vi "Instrument Manager Loop.vi"(8 "System Control":refnum<queue>, 11 "Instrument Manager":refnum<queue>) -> (0 "error out":errorcluster)   [LabVIEW 2020, in "Omega Platinum Series Plugin.lvlib" / "Instrument Manager.lvlib"]
uses:
  Instrument Manager/Instrument Manager.lvlib
  support/Message Queue/Message Cluster.ctl
  Instrument Manager/Instrument State.ctl
  <vilib>/Utility/error.llb/Error Cluster From Error Code.vi
  <vilib>/ErrorRing/Error Ring.xnode
  support/Message Queue/Message Queue.lvlib
  Omega Platinum Series Plugin.lvlib
  <instrlib>/Omega Platinum Series/Omega Platinum Series.lvlib
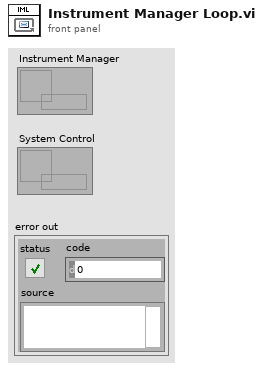
[diagram p1: front panel]
types:
  T1 = typedef "Omega Platinum Series Plugin.lvlib/Instrument Manager.lvlib/Instrument State.ctl" = cluster{"VISA Resource":refnum<visa-resource-name>, "Setpoint":dbl, "Running":bool, "Running Since":timestamp, "Data Point":cluster{"Time Stamp":timestamp, "Value":dbl}, "Sampling Rate (sec/sample)":dbl}
  T2 = typedef "Omega Platinum Series.lvlib/System State.ctl" = enum16{"LOAD", "IDLE", "INPUT_ADJUST", "CONTROL_ADJUST", "MODIFY", "WAIT", "RUN", "STANDBY", "STOP", "PAUSE", "FAULT", "SHUTDOWN", "AUTOTUNE"}
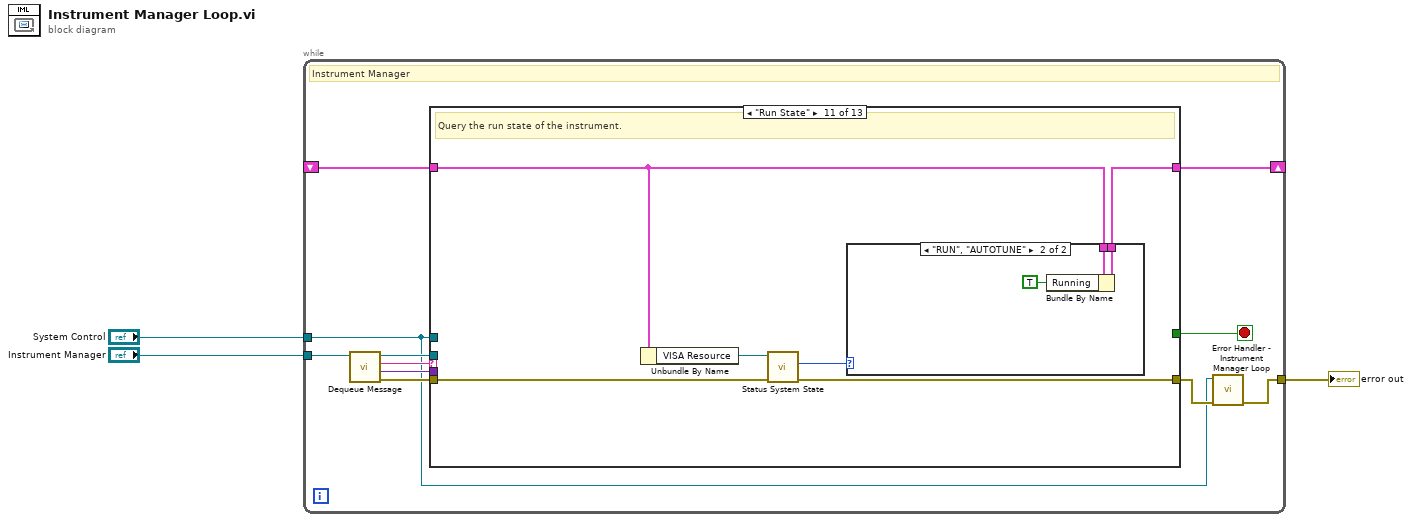
[diagram p0: block diagram]
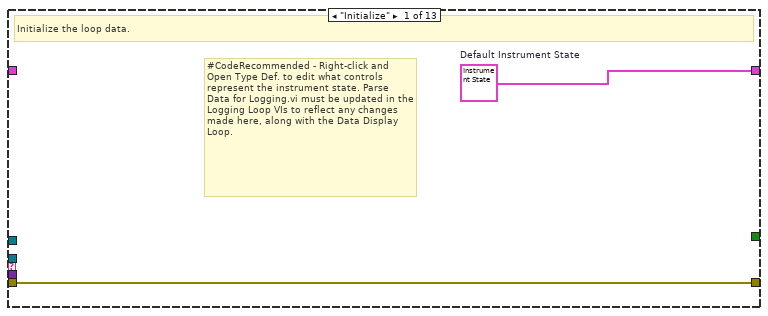
[diagram p2: hidden frame]
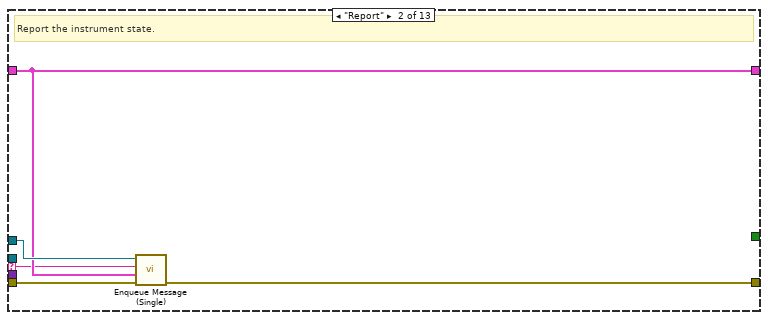
[diagram p3: hidden frame]
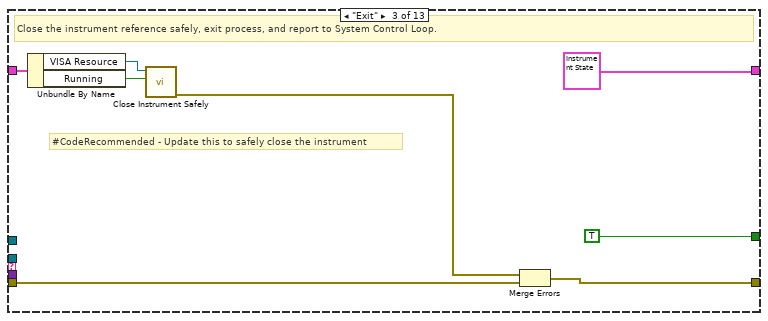
[diagram p4: hidden frame]
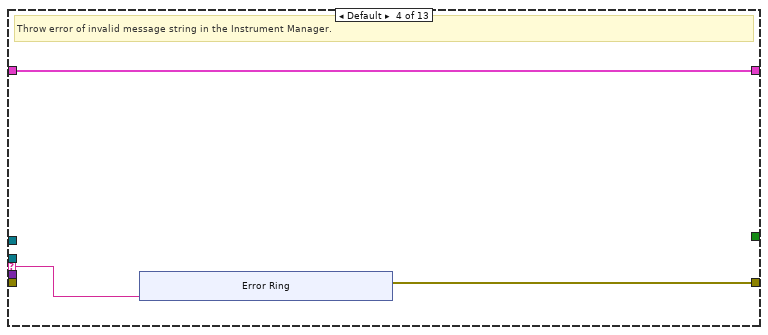
[diagram p5: hidden frame]
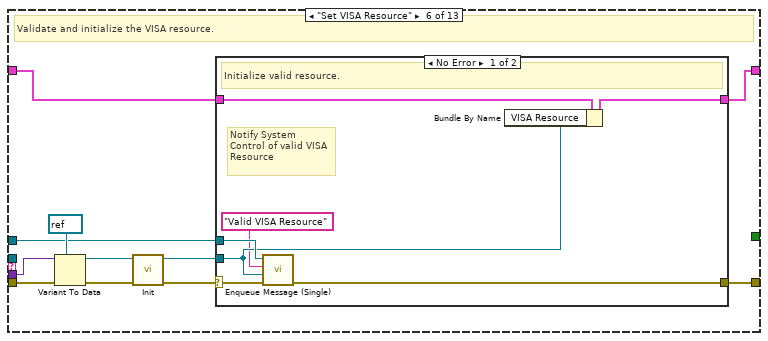
[diagram p7: hidden frame]
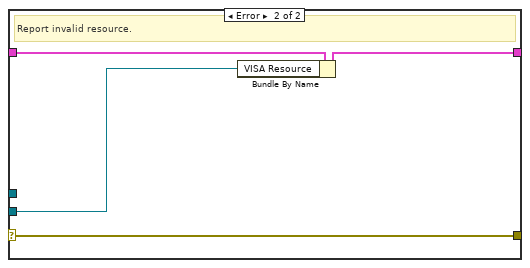
[diagram p8: hidden frame]
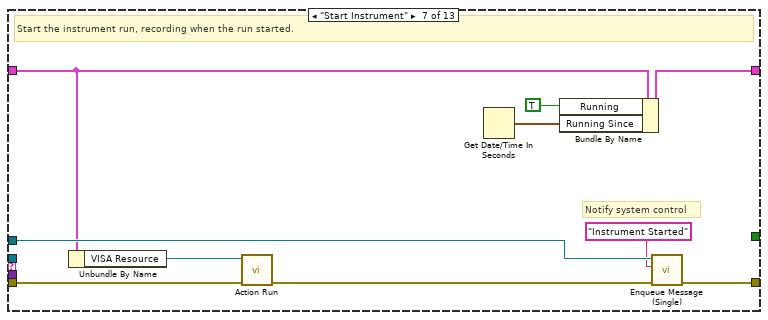
[diagram p9: hidden frame]
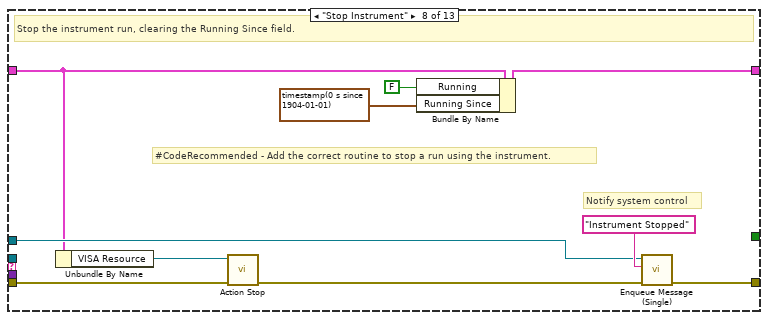
[diagram p10: hidden frame]
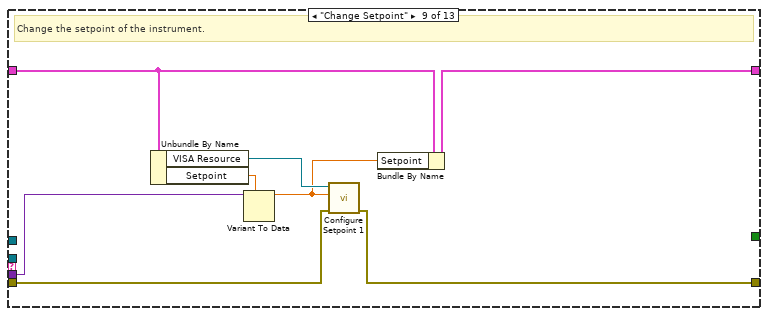
[diagram p11: hidden frame]
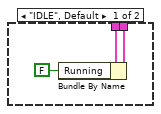
[diagram p13: hidden frame]
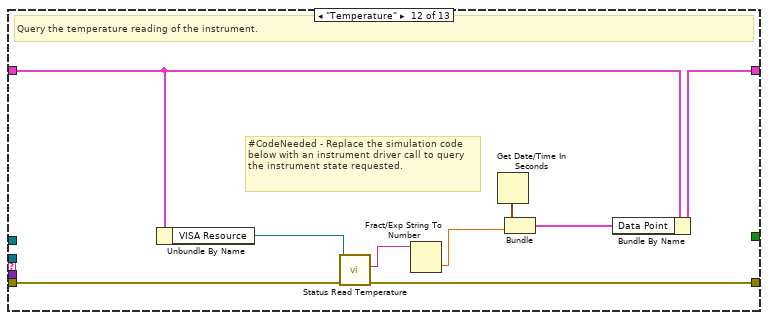
[diagram p14: hidden frame]
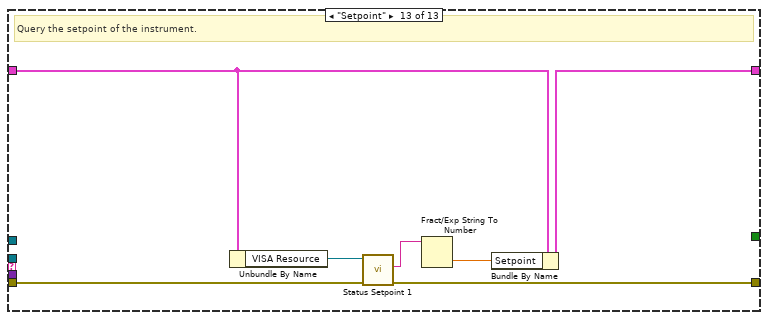
[diagram p15: hidden frame]
diagram:
  n1 = while {
    tunnel: "Instrument Manager" -> [w14]
    tunnel: "System Control" -> [w5]
    tunnel: [w8] -> w1
    shift-right: [w7] -> _
    shift-left: _ -> [w4]
    stop <- w6 stop-if-true
    # "Instrument Manager"
    n2 = call "Dequeue Message.vi"("Message Queue"=w14) -> ("error out"=w10:errorcluster, "Message Data"=w11:variant, "Message"=w13:string, "dup Message Queue"=w12:refnum<queue>)  [unwired: 7 in]
    n3 = case shown="\"Run State\"" w13 {
      selector: w13 -> [_ w17 _ w31 _ _ _ _ _ _ _ _ _]
      tunnel: w12 -> [_ _ _ _ _ _ _ _ _ _ _ _ _]
      tunnel: w5 -> [_ w20 _ _ _ w42 w72 w81 _ _ _ _ _]
      tunnel: w11 -> [_ _ _ _ _ w49 _ _ w90 _ _ _ _]
      tunnel: w10 -> [w15 w21 w24 _ w40 w48 w65 w76 w87 w93 w99 w109 w121]
      tunnel: [w15 w19 w23 w30 w40 w52 w73 w83 w86 w93 w98 w108 w120] -> w9
      tunnel: w4 -> [_ w18 w29 w32 w41 w51 w67 w74 w89 w92 w94 w111 w119]
      tunnel: [w16 w18 T1 {"VISA Resource"="", "Setpoint"=0.0, "Running"=FALSE, "Running Since"=timestamp(0 s since 1904-01-01), "Data Point"={"Time Stamp"=timestamp(0 s since 1904-01-01), "Value"=0.0}, "Sampling Rate (sec/sample)"=0.0} w32 w41 w50 w70 w80 w91 w92 w95 w114 w117] -> w7
      tunnel: [_ _ TRUE _ _ _ _ _ _ _ _ _ _] -> w6
      frame "Initialize" {
        w16 = T1 {"VISA Resource"="", "Setpoint"=0.0, "Running"=FALSE, "Running Since"=timestamp(0 s since 1904-01-01), "Data Point"={"Time Stamp"=timestamp(0 s since 1904-01-01), "Value"=0.0}, "Sampling Rate (sec/sample)"=0.0}  # Default Instrument State
        # "#CodeRecommended - Right-click and Open Type Def. to edit what controls represent the instrument state. Parse Data for Logging.vi must be updated in the Logging Loop VIs to reflect any changes made here, along with the Data Display Loop."
        # "Initialize the loop data."
      }
      frame "Report" {
        # "Report the instrument state."
        n4 = call "Enqueue Message (Single).vi"("error in (no error)"=w21, "Message Data"=w18, "Message"=w17, "Message Queue"=w20) -> ("error out"=w19:errorcluster)  [unwired: 6 in, 1 out]
      }
      frame "Exit" {
        # "#CodeRecommended - Update this to safely close the instrument"
        # "Close the instrument reference safely, exit process, and report to System Control Loop."
        n5 = Unbundle By Name(w29) -> ("VISA Resource"=w27:refnum<visa-resource-name>, "Running"=w28:bool)
        n6 = call "Close Instrument Safely.vi"("Running (F)"=w28, "VISA Refnum in"=w27) -> ("error out"=w22:errorcluster)  [unwired: 9 in]
        n7 = Merge Errors(w22, w24) -> (w23:errorcluster)
      }
      frame Default {
        # "Throw error of invalid message string in the Instrument Manager."
        n8 = xnode "Error Ring"("parameter 0"=w31) -> ("error out"=w30:errorcluster)
      }
      frame "--- Copy This Frame ---" {
        # "Copy this frame and add responses to instrument specific messages."
      }
      frame "Set VISA Resource" {
        # "Validate and initialize the VISA resource."
        n9 = Variant To Data(error in=w48, type=refnum<visa-resource-name> refnum, Variant=w49) -> (data=w46:refnum<visa-resource-name>, error out=w47:errorcluster)
        n10 = call "Init.vi"("error in (no error)"=w47, "VISA resource in"=w46) -> ("error out"=w43:errorcluster, "VISA resource out"=w44:refnum<visa-resource-name>)  [unwired: 8 in]
        n11 = case shown="No Error" w43 {
          selector: w43 -> [w58 w60]
          tunnel: w44 -> [w55 w61]
          tunnel: [w57 w60] -> w52
          tunnel: w51 -> [w59 w63]
          tunnel: [w53 w62] -> w50
          tunnel: w42 -> [w56 _]
          frame No Error {
            # "Notify System Control of valid VISA Resource"
            # "Initialize valid resource."
            n12 = call "Enqueue Message (Single).vi"("error in (no error)"=w58, "Message Data"=w55, "Message"="Valid VISA Resource", "Message Queue"=w56) -> ("error out"=w57:errorcluster)  [unwired: 6 in, 1 out]
            n13 = Bundle By Name(cluster=w59, "VISA Resource"=w55) -> (w53:T1)
          }
          frame Error {
            # "Report invalid resource."
            n14 = Bundle By Name(cluster=w63, "VISA Resource"=w61) -> (w62:T1)
          }
        }
      }
      frame "Start Instrument" {
        # "Notify system control"
        # "Start the instrument run, recording when the run started."
        n15 = Unbundle By Name(w67) -> ("VISA Resource"=w66:refnum<visa-resource-name>)
        n16 = call <instrlib>:"Action Run.vi"("error in (no error)"=w65, "VISA resource name (in)"=w66) -> ("error out"=w64:errorcluster)  [unwired: 7 in, 2 out]
        n17 = Get Date/Time In Seconds() -> (seconds since 1Jan1904=w68:timestamp)
        n18 = Bundle By Name(cluster=w67, "Running"=TRUE, "Running Since"=w68) -> (w70:T1)
        n19 = call "Enqueue Message (Single).vi"("error in (no error)"=w64, "Message"="Instrument Started", "Message Queue"=w72) -> ("error out"=w73:errorcluster)  [unwired: 7 in, 1 out]
      }
      frame "Stop Instrument" {
        # "Notify system control"
        # "#CodeRecommended - Add the correct routine to stop a run using the instrument."
        # "Stop the instrument run, clearing the Running Since field."
        n20 = Unbundle By Name(w74) -> ("VISA Resource"=w77:refnum<visa-resource-name>)
        n21 = call <instrlib>:"Action Stop.vi"("error in (no error)"=w76, "VISA resource name (in)"=w77) -> ("error out"=w75:errorcluster)  [unwired: 7 in, 2 out]
        n22 = Bundle By Name(cluster=w74, "Running"=FALSE, "Running Since"=timestamp(0 s since 1904-01-01)) -> (w80:T1)
        n23 = call "Enqueue Message (Single).vi"("error in (no error)"=w75, "Message"="Instrument Stopped", "Message Queue"=w81) -> ("error out"=w83:errorcluster)  [unwired: 7 in, 1 out]
      }
      frame "Change Setpoint" {
        # "Change the setpoint of the instrument."
        n24 = Unbundle By Name(w89) -> ("VISA Resource"=w85:refnum<visa-resource-name>, "Setpoint"=w88:dbl)
        n25 = Variant To Data(type=w88, Variant=w90) -> (data=w84:dbl)  [unwired: 1 in, 1 out]
        n26 = call <instrlib>:"Configure Setpoint 1.vi"("error in (no error)"=w87, "Setpoint value"=w84, "VISA resource name (in)"=w85) -> ("error out"=w86:errorcluster)  [unwired: 6 in, 2 out]
        n27 = Bundle By Name(cluster=w89, "Setpoint"=w84) -> (w91:T1)
      }
      frame "--- Copy for Get State Messages ---" {
        # "#CodeNeeded - Use the Bundle by Name function to bundle the new state value into the Instrument State cluster."
        # "#CodeNeeded - Add instrument driver call to query the instrument state requested"
        # "Duplicate this case for messages cases that will query the instrument state."
      }
      frame "Run State" {
        # "Query the run state of the instrument."
        n28 = Unbundle By Name(w94) -> ("VISA Resource"=w97:refnum<visa-resource-name>)
        n29 = call <instrlib>:"Status System State.vi"("error in (no error)"=w99, "VISA resource name (in)"=w97) -> ("error out"=w98:errorcluster, "System State"=w96:T2)  [unwired: 7 in, 1 out]
        n30 = case shown="\"RUN\", \"AUTOTUNE\"" w96 {
          tunnel: w94 -> [w101 w105]
          tunnel: [w102 w104] -> w95
          frame "IDLE", Default {
            n31 = Bundle By Name(cluster=w101, "Running"=FALSE) -> (w102:T1)
          }
          frame "RUN", "AUTOTUNE" {
            n32 = Bundle By Name(cluster=w105, "Running"=TRUE) -> (w104:T1)
          }
        }
      }
      frame "Temperature" {
        # "#CodeNeeded - Replace the simulation code below with an instrument driver call to query the instrument state requested."
        # "Query the temperature reading of the instrument."
        n33 = Unbundle By Name(w111) -> ("VISA Resource"=w110:refnum<visa-resource-name>)
        n34 = call <instrlib>:"Status Read Temperature.vi"("error in (no error)"=w109, "VISA resource name (in)"=w110) -> ("error out"=w108:errorcluster, "Temperature"=w107:string)  [unwired: 7 in, 1 out]
        n35 = Fract/Exp String To Number(string=w107) -> (number=w106:dbl)  [unwired: 3 in, 1 out]
        n36 = Get Date/Time In Seconds() -> (seconds since 1Jan1904=w113:timestamp)
        n37 = Bundle("seconds since 1Jan1904"=w113, w106) -> (w112:cluster{"seconds since 1Jan1904":timestamp, dbl})  [unwired: 1 in]
        n38 = Bundle By Name(cluster=w111, "Data Point"=w112) -> (w114:T1)
      }
      frame "Setpoint" {
        # "Query the setpoint of the instrument."
        n39 = Unbundle By Name(w119) -> ("VISA Resource"=w118:refnum<visa-resource-name>)
        n40 = call <instrlib>:"Status Setpoint 1.vi"("error in (no error)"=w121, "VISA resource name (in)"=w118) -> ("error out"=w120:errorcluster, "Setpoint 1"=w116:string)  [unwired: 7 in, 1 out]
        n41 = Fract/Exp String To Number(string=w116) -> (number=w115:dbl)  [unwired: 3 in, 1 out]
        n42 = Bundle By Name(cluster=w119, "Setpoint"=w115) -> (w117:T1)
      }
    }
    n43 = call "Error Handler - Instrument Manager Loop.vi"("error in (no error)"=w9, "Message Queue"=w5) -> ("dup error in"=w8:errorcluster)  [unwired: 8 in, 1 out]
  }
  "error out" <- w1
